vi "Example.vi"() -> ()   [LabVIEW 2013]
uses:
  StellarNetSpectrometer.lvclass
panel:
  in  "Settings":T1={"Integration Time (ms)"=80, "Temp  Compensation "=FALSE, "Optical Smoothing Level"=0, "Number of Scans to Average"=1, "Digitizer Clock Rate Setting"=3} {"Digitizer Clock Rate Setting" min=1 max=3; "Number of Scans to Average" min=1 max=10000 step=1; "Optical Smoothing Level" min=0 max=4 step=1}
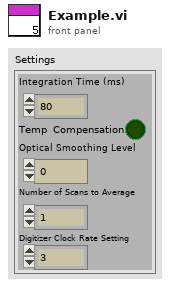
[diagram p1: front panel]
types:
  T1 = cluster{"Integration Time (ms)":i32, "Temp  Compensation ":bool, "Optical Smoothing Level":i32, "Number of Scans to Average":i32, "Digitizer Clock Rate Setting":i32}
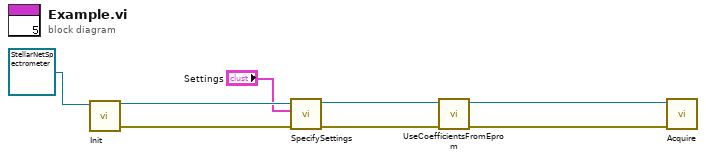
[diagram p0: block diagram]
diagram:
  n1 = call-dynamic "Init.vi"("StellarNetSpectrometer in"=refnum<class "StellarNetSpectrometer.lvclass"> refnum ("StellarNetSpectrometer.lvclass")) -> ("error out"=w6:errorcluster, "StellarNetSpectrometer out"=w7:refnum<class "StellarNetSpectrometer.lvclass">)  [unwired: 9 in]
  n2 = call-dynamic "SpecifySettings.vi"("error in"=w6, "Settings"="Settings", "StellarNetSpectrometer in"=w7) -> ("error out"=w3:errorcluster, "StellarNetSpectrometer out"=w4:refnum<class "StellarNetSpectrometer.lvclass">)  [unwired: 7 in]
  n3 = call-dynamic "UseCoefficientsFromEprom.vi"("error in"=w3, "StellarNetSpectrometer in"=w4) -> ("error out"=w2:errorcluster, "StellarNetSpectrometer out"=w1:refnum<class "StellarNetSpectrometer.lvclass">)  [unwired: 8 in]
  n4 = call-dynamic "Acquire.vi"("error in"=w2, "StellarNetSpectrometer in"=w1) -> ()  [unwired: 8 in, 2 out]
